vi "运维调试_总磷总氮.vi"() -> ()   [LabVIEW 2016, in "斯坦道氨氮.lvlib"]
uses:
  <vilib>/Utility/miscctls.llb/LVPointTypeDef.ctl
  <vilib>/Plasmionique/MB Master/MB_Master/MB_Master.lvclass
  <vilib>/ptbypt/NI_PtbyPt.lvlib
panel:
  out "seconds since 1Jan1904 2":timestamp
  out "seconds since 1Jan1904":timestamp
  in  "周期设置":bool
  in  "流程操作":bool
  out "消解压力":sgl format="%#.2f kPa"
  out "权限等级":string
  out "总步数":i32
  out "滑动杆":u8(slide) caption="测试进度" scale=0.0..100.0
  out "试剂余量显示":sgl[][](graph)
  in  "仪器校准":bool
  in  "参数查询":bool
  out "简易步骤名称":string
  in  "温度曲线":bool
  in  "试剂余量":bool
  in  "灯值调整":bool
  out "固件版本号":string
  out "模块版本号":string
  out "注射器温度":sgl format="%#.2f ℃"
  out "消解温度":sgl format="%#.2f ℃"
  out "ADC":sgl
  out "F3":sgl format="%#.6f"
  out "F2":sgl format="%#.6f"
  out "F1":sgl format="%#.6f"
  out "F0":sgl format="%#.6f"
  out "运行状态":T1 {"数据时间:" format="%<%y/%m/%d %H:%M:%S>T"; "仪器时间:" format="%<%y/%m/%d %H:%M:%S>T"}
  in  "单选按钮":T2=enum."总氮"
  in  "布尔":bool
  in  "外设固件":bool
  out "字符串 2":string
  in  "数组":string[](array[string])
  in  "返回":bool
  in  "参数设置":bool
  out "集成报警信息":string
  in  "停止":bool
  in  "手动启动":bool
  in  "调试":bool
  out "多列列表框":i32(listbox)
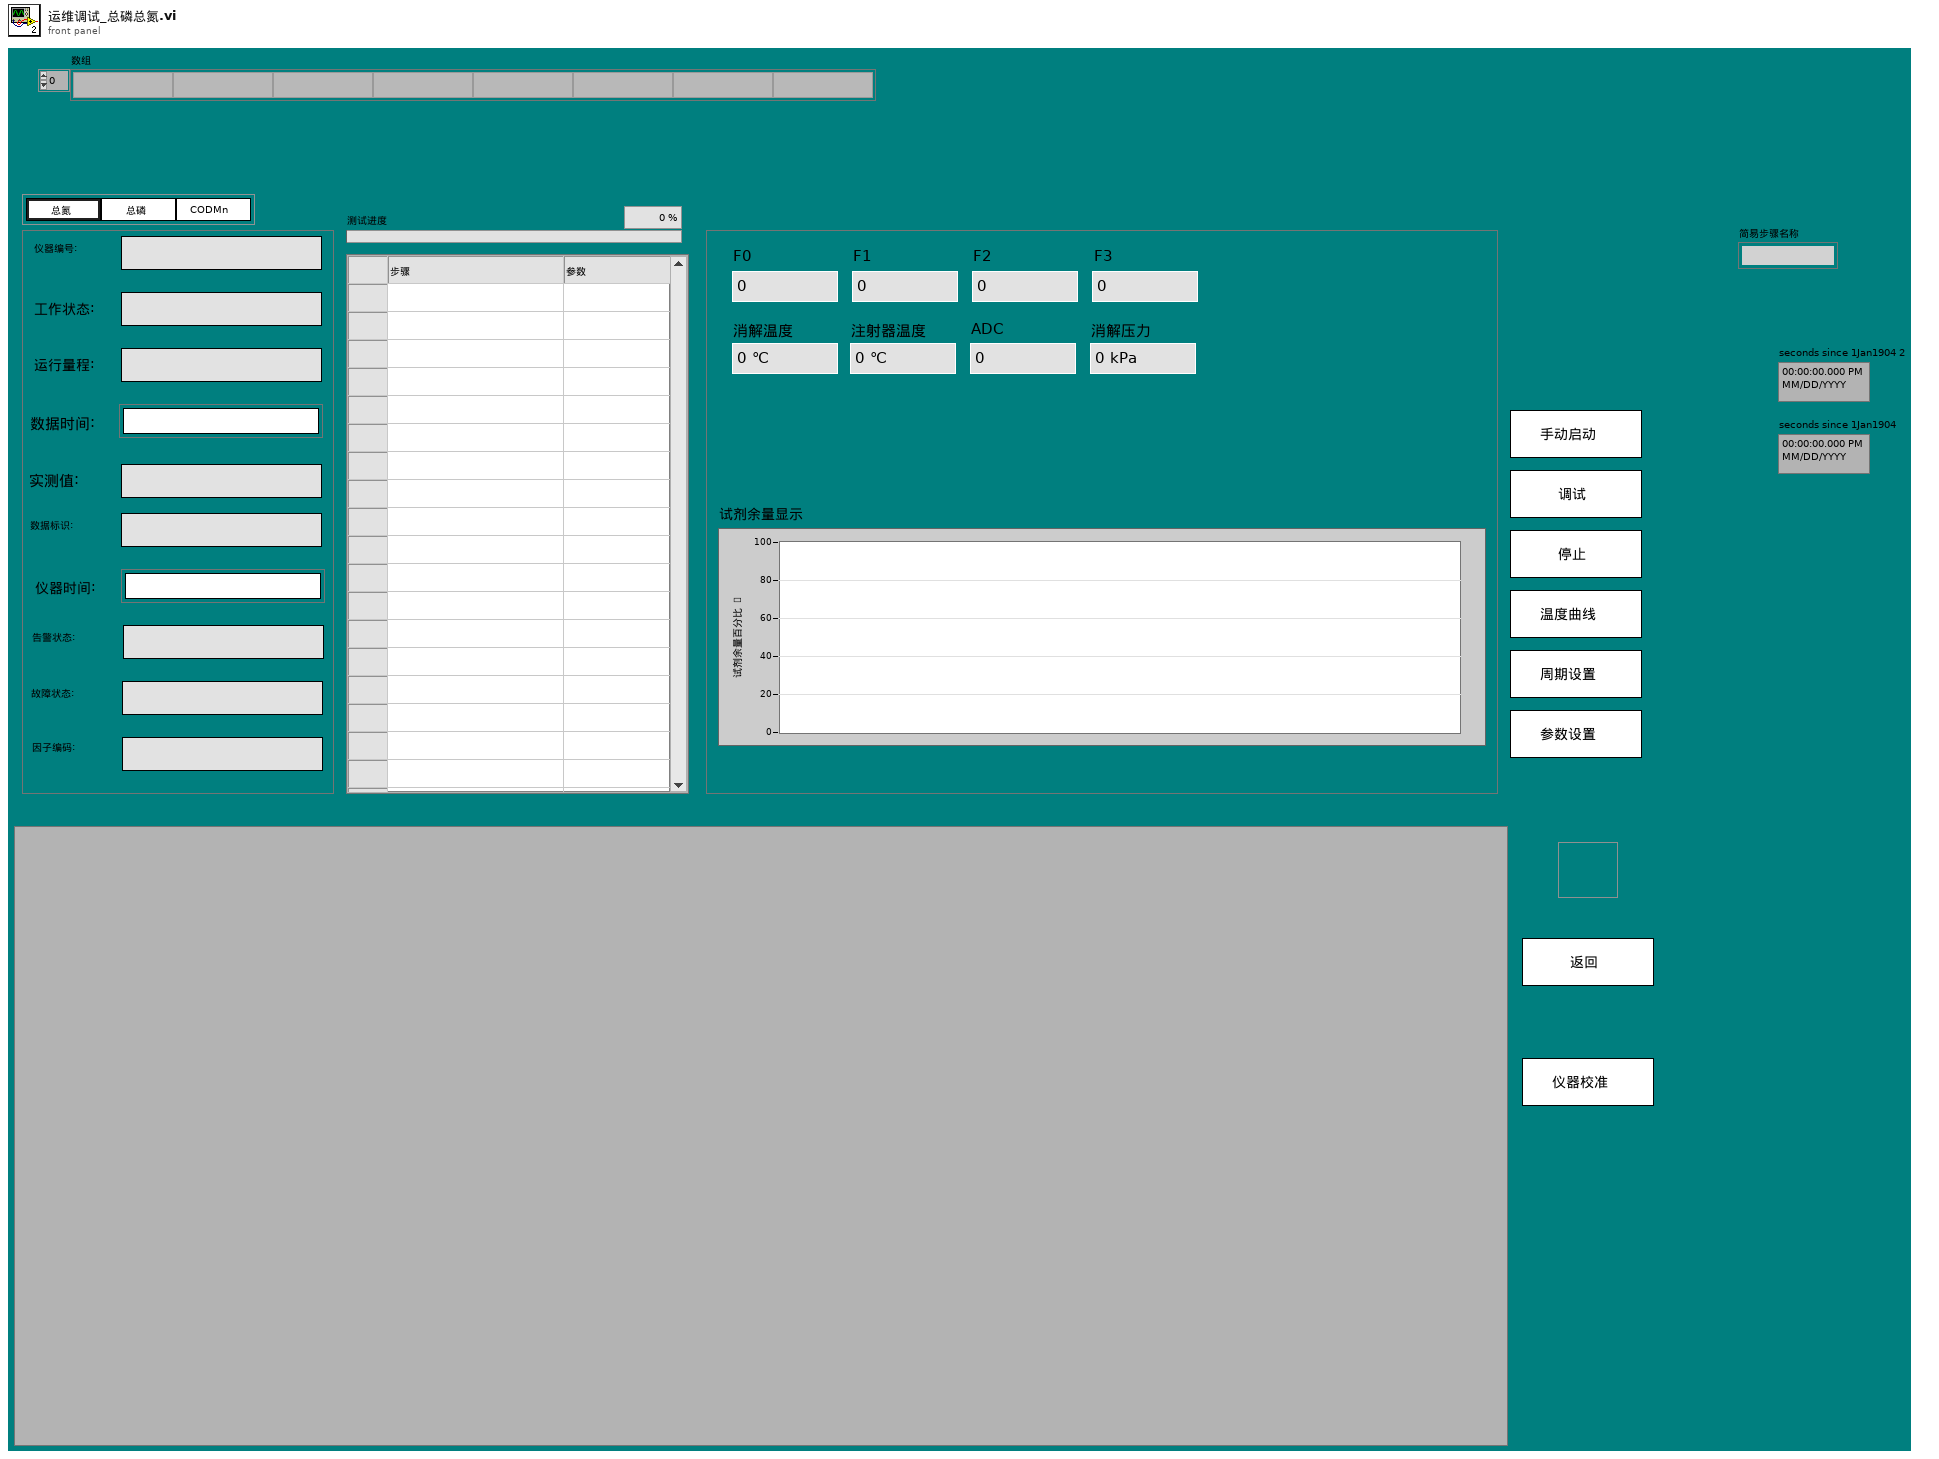
[diagram p1: front panel]
types:
  T1 = cluster{"仪器编号:":string, "工作状态:":string, "运行量程: ":string, "数据时间:":timestamp, "实测值:":string, "数据标识: ":string, "仪器时间:":timestamp, "告警状态: ":string, "故障状态:  ":string, "因子编码:":string}
  T2 = typedef "斯坦道氨氮.lvlib/启动参数显示控件.ctl" = enum32{"COD", "氨氮", "总氮", "总磷", "磷酸盐", "硝氮", "亚硝氮", "硅酸盐", "硫化物", "氟化物", "CODMn"}
  T3 = cluster{"Major":u16, "Minor":u16, "Fix":u16, "Build":u16}
  T4 = typedef "斯坦道总磷总氮.lvlib/启动参数显示控件.ctl" = enum32{"COD", "氨氮", "总氮", "总磷", "磷酸盐", "硝氮", "亚硝氮", "硅酸盐", "硫化物", "氟化物", "CODMn"}
  T5 = typedef "LVPointTypeDef.ctl" = cluster{"Horizontal":i16, "Vertical":i16}
  T6 = cluster{"系统时间":timestamp, "工作状态":u16, "测量模式":enum16{"待机", "连续模式", "周期模式", "定点模式", "受控模式", "手动模式"}, "告警代码":u16, "故障代码":u16, "日志代码":u16, "软件版本":u16, "F0":sgl, "F1":sgl, "F2":sgl, "F3":sgl, "T":sgl, "H":sgl, "id":u16, "flowid":u16, "量程":u16, "总磷控温温度1":sgl, "营养盐控温温度2":sgl, "ADC":sgl}
  T7 = typedef "Alarm interface.lvlib/报警短信语音交互.ctl" = cluster{"参数":string, "元器件":string, "故障现象":string, "code":string, "platform_alarm_code":string, "solutionList":cluster{"reason":string, "solution":string}[]}
  T8 = typedef "SingleStepTestV3.lvlib/SingleStepTestV3.lvclass/仪器版本.ctl" = enum16{"A版", "B版", "A1版"}
  T9 = cluster{"因子编码":u32, "单位":u16, "标样参考值":sgl, "水样数据时间":timestamp, "水样实测值":sgl, "水样数据标识":string, "标样数据时间":timestamp, "标样实测值":sgl, "标样数据标识":string, "空白数据时间":timestamp, "空白实测值":sgl, "空白数据标识":string, "零点核查数据时间":timestamp, "零点核查实测值":sgl, "零点核查数据标识":string, "跨度核查数据时间":timestamp, "跨度核查实测值":sgl, "跨度核查数据标识":string, "加标回收数据时间":timestamp, "加标回收实测值":sgl, "加标回收数据标识":string, "平行样数据时间":timestamp, "平行样实测值":sgl, "平行样数据标识":string, "F0":sgl, "F1":sgl, "F2":sgl, "F3":sgl, "F4":sgl, "F5":sgl, "F6":sgl, "F7":sgl, "温度":sgl, "湿度":sgl, "X值":sgl, "fidrange":u16, "X1值":sgl}[]
  T10 = cluster{"因子编码":u32, "单位":u16, "标样参考值":sgl, "水样数据时间":timestamp, "水样实测值":sgl, "水样数据标识":string, "标样数据时间":timestamp, "标样实测值":sgl, "标样数据标识":string, "空白数据时间":timestamp, "空白实测值":sgl, "空白数据标识":string, "零点核查数据时间":timestamp, "零点核查实测值":sgl, "零点核查数据标识":string, "跨度核查数据时间":timestamp, "跨度核查实测值":sgl, "跨度核查数据标识":string, "加标回收数据时间":timestamp, "加标回收实测值":sgl, "加标回收数据标识":string, "平行样数据时间":timestamp, "平行样实测值":sgl, "平行样数据标识":string, "F0":sgl, "F1":sgl, "F2":sgl, "F3":sgl, "F4":sgl, "F5":sgl, "F6":sgl, "F7":sgl, "温度":sgl, "湿度":sgl, "X值":sgl, "fidrange":u16, "X1值":sgl}
  T11 = typedef "TimingControl.lvlib/TimingControl.lvclass/国标控制命令.ctl" = enum16{"启动测量", "标样核查", "零点核查", "跨度核查", "空白测试", "平行样测试", "加标回收", "空白校准", "标样校准", "初始化（清洗）", "停止测试", "仪器重启", "校时", "模式设置", "测量间隔设置"}
  T12 = typedef "TimingControl.lvlib/TimingControl.lvclass/测量参数.ctl" = u16
  T13 = enum32{"Bad", "Idle", "Run top level", "Running"}
  T14 = enum16{"空闲", "水样测试", "标样核查", "零点核查", "跨度核查", "空白测试", "平行样测试", "加标回收", "空白校准", "标样校准", "初始化（清洗）"}
  T15 = cluster{"站号":u16, "量程切换":enum32{"H", "L", "AUTO"}, "控制命令":enum16{"启动测量", "标样核查", "零点核查", "跨度核查", "空白测试", "平行样测试", "加标回收", "空白校准", "标样校准", "初始化（清洗）", "停止测试", "仪器重启", "校时", "模式设置", "测量间隔设置"}, "模式设置":enum16{"待机", "连续模式", "周期模式", "定点模式", "受控模式", "手动模式"}, "测量间隔":u16}
  T16 = cluster{"时间标识":timestamp, "设备":string, "日志信息":string, "流程参数":string}
  T17 = typedef "LVRowAndColumnUnsignedTypeDef.ctl" = cluster{"Row":u32, "Column":u32}
  T18 = typedef "操作日志字段定义.ctl" = cluster{"时间":timestamp, "参数":string, "日志信息":string, "流程参数":string}
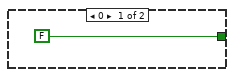
[diagram p4: hidden frame]
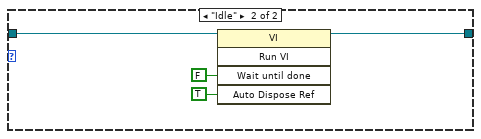
[diagram p8: hidden frame]
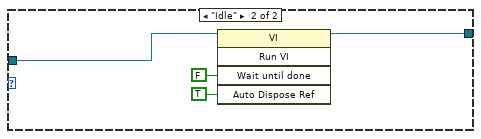
[diagram p9: hidden frame]
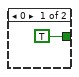
[diagram p11: hidden frame]
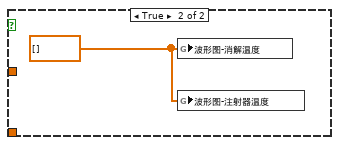
[diagram p12: hidden frame]
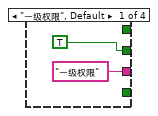
[diagram p14: hidden frame]
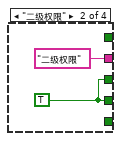
[diagram p15: hidden frame]
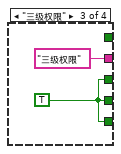
[diagram p16: hidden frame]
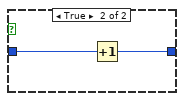
[diagram p18: hidden frame]
diagram:
  n1 = flat-sequence {
    tunnel: [w27] -> w18
    tunnel: w18 -> [w39]
    tunnel: [w39] -> w17
    tunnel: w17 -> [w64]
    tunnel: [w155] -> w19
    tunnel: [errorcluster {"status"=FALSE, "code"=0, "source"=""} ("错误输入（无错误）")] -> w8
    tunnel: [errorcluster {"status"=FALSE, "code"=0, "source"=""} ("错误输入（无错误）")] -> w7
    tunnel: [w152] -> w5
    tunnel: [errorcluster {"status"=FALSE, "code"=0, "source"=""} ("error out")] -> w4
    tunnel: [errorcluster {"status"=FALSE, "code"=0, "source"=""} ("错误输入（无错误）")] -> w3
    frame #0 {
      n2 = control-ref of="本VI"() -> (w29:refnum<vi>)
      n3 = control-ref of="本VI"() -> (w38:refnum<vi>)
      n4 = property class="VI"(reference=w29) -> ("Library"=w30:refnum<vi>)  [unwired: 1 in, 2 out]
      n5 = property class="VI"(reference=w38) -> ("Library.Version"=w37:T3)  [unwired: 1 in, 2 out]
      n6 = global read "VAR总磷总氮全局变量.vi" "初始化"() -> (w26:bool)
      n7 = case shown="假" w26 {
        frame False {
          n8 = call "配置初始化.vi"() -> ()  [unwired: 11 in, 1 out]
        }
        frame True {
        }
      }
      n9 = property class="Library"(reference=w30) -> ("Path"=w28:path)  [unwired: 1 in, 2 out]
      n10 = Unbundle By Name(w37) -> ("Major"=w35:u16, "Minor"=w34:u16, "Fix"=w33:u16, "Build"=w32:u16)
      n11 = call "新建通讯互斥锁.vi"() -> ()  [unwired: 11 in, 1 out]
      n12 = Format Into String(format string="模块版本号：%d.%d.%d.%d" ("格式字符串"), w35, w34, w33, w32) -> (resulting string=→"模块版本号":string)  [unwired: 2 in, 1 out]
      n13 = call <vilib>:"Get File Extension.vi"("file"=w28) -> ("filename without extension"=w27:string)  [unwired: 6 in, 4 out]
    }
    frame #1 {
      n14 = global read "总磷总氮断电保存全局变量.vi" "IP"() -> (w43:string)
      n15 = global read "总磷总氮断电保存全局变量.vi" "VISA Resource"() -> (w40:refnum<visa-resource-name>)
      n16 = Empty String/Path?(string/path=w43) -> (empty?=w42:bool)
      n17 = Empty String/Path?(string/path=w40) -> (empty?=w41:bool)
      n18 = case shown="真" w42 {
        tunnel: w39 -> [_ w55]
        frame False {
        }
        frame True {
          n19 = case shown="\"斯坦道CODMn\"" w55 {
            tunnel: [w56 "192.168.1.203" ("IP") "192.168.1.202" ("IP") "192.168.1.202" ("IP") "192.168.1.203" ("IP") "192.168.1.204" ("IP") "192.168.1.205" ("IP") "192.168.1.201" ("IP")] -> w54
            frame Default {
              n20 = global read "总磷总氮断电保存全局变量.vi" "IP"() -> (w56:string)
            }
            frame "斯坦道总磷总氮" {
            }
            frame "斯坦道氨氮" {
            }
            frame "斯坦道氨氮总磷" {
            }
            frame "斯坦道总磷" {
            }
            frame "斯坦道总氮" {
            }
            frame "斯坦道CODcr" {
            }
            frame "斯坦道CODMn" {
            }
          }
          n21 = global write "总磷总氮断电保存全局变量.vi" "IP"(w54) -> ()
        }
      }
      n22 = case shown="真" w41 {
        tunnel: w39 -> [_ w45]
        frame False {
        }
        frame True {
          n23 = case shown="\"斯坦道CODMn\"" w45 {
            tunnel: [w46 "COM5" ("IP") "COM7" ("IP") "COM7" ("IP") "COM5" ("IP") "COM10" ("IP") "COM9" ("IP") "COM4" ("IP")] -> w44
            frame Default {
              n24 = global read "总磷总氮断电保存全局变量.vi" "VISA Resource"() -> (w46:refnum<visa-resource-name>)
            }
            frame "斯坦道总磷总氮" {
            }
            frame "斯坦道氨氮" {
            }
            frame "斯坦道氨氮总磷" {
            }
            frame "斯坦道总磷" {
            }
            frame "斯坦道总氮" {
            }
            frame "斯坦道CODcr" {
            }
            frame "斯坦道CODMn" {
            }
          }
          n25 = global write "总磷总氮断电保存全局变量.vi" "VISA Resource"(w44) -> ()
        }
      }
    }
    frame #2 {
      n26 = global read "model config var.vi" "启动队列名称"() -> (w66:cluster{"String":string, "Value":u16}[])
      n27 = Empty Array?(array=w66) -> (empty?=w65:bool)
      n28 = case shown="真" w65 {
        tunnel: w64 -> [_ w67]
        frame False {
        }
        frame True {
          n29 = global read "总磷总氮断电保存全局变量.vi" "PORT"() -> (w73:string)
          n30 = Decimal String To Number(string=w73) -> (number=w72:i32)  [unwired: 2 in, 1 out]
          n31 = global read "总磷总氮断电保存全局变量.vi" "MB通信方式选择"() -> (w71:enum16{"串口", "TCP"})
          n32 = global read "总磷总氮断电保存全局变量.vi" "VISA Resource"() -> (w70:refnum<visa-resource-name>)
          n33 = global read "总磷总氮断电保存全局变量.vi" "IP"() -> (w74:string)
          n34 = call "获取启动参数.vi"("MB通信方式选择"=w71, "Port (502)"=w72, "IP Address"=w74, "VISA Resource"=w70) -> ("error out"=w69:errorcluster, "数组"=w68:cluster{"String":string, "Value":u16}[])  [unwired: 6 in]
          n35 = flat-sequence {
            tunnel: w69 -> [w76]
            tunnel: w68 -> [w75]
            tunnel: w67 -> [w78]
            frame #0 {
              n36 = case shown="无错误" w76 {
                tunnel: w75 -> [w77 _]
                frame No Error {
                  n37 = global write "model config var.vi" "启动队列名称"(w77) -> ()
                }
                frame Error {
                }
              }
            }
            frame #1 {
              n38 = global read "model config var.vi" "启动队列名称"() -> (w80:cluster{"String":string, "Value":u16}[])
              n39 = Empty Array?(array=w80) -> (empty?=w79:bool)
              n40 = case shown="真" w79 {
                tunnel: w78 -> [_ w81]
                frame False {
                }
                frame True {
                  n41 = case shown="\"斯坦道CODmn\"" w81 {
                    frame Default {
                    }
                    frame "斯坦道总磷总氮" {
                      n42 = global write "model config var.vi" "启动队列名称"(cluster{"String":string, "Value":u16}[] [{"String"="总氮", "Value"=2}, {"String"="总磷", "Value"=1}] ("启动队列名称")) -> ()
                    }
                    frame "斯坦道氨氮" {
                      n43 = global write "model config var.vi" "启动队列名称"(cluster{"String":string, "Value":u16}[] [{"String"="氨氮", "Value"=3}] ("启动队列名称")) -> ()
                    }
                    frame "斯坦道氨氮总磷" {
                      n44 = global write "model config var.vi" "启动队列名称"(cluster{"String":string, "Value":u16}[] [{"String"="氨氮", "Value"=3}, {"String"="总磷", "Value"=1}] ("启动队列名称")) -> ()
                    }
                    frame "斯坦道总磷" {
                      n45 = global write "model config var.vi" "启动队列名称"(cluster{"String":string, "Value":u16}[] [{"String"="总磷", "Value"=1}] ("启动队列名称")) -> ()
                    }
                    frame "斯坦道总氮" {
                      n46 = global write "model config var.vi" "启动队列名称"(cluster{"String":string, "Value":u16}[] [{"String"="总氮", "Value"=2}] ("启动队列名称")) -> ()
                    }
                    frame "斯坦道CODcr" {
                      n47 = global write "model config var.vi" "启动队列名称"(cluster{"String":string, "Value":u16}[] [{"String"="CODcr", "Value"=22}] ("启动队列名称")) -> ()
                    }
                    frame "斯坦道氟化物" {
                      n48 = global write "model config var.vi" "启动队列名称"(cluster{"String":string, "Value":u16}[] [{"String"="氟化物", "Value"=50}] ("启动队列名称")) -> ()
                    }
                    frame "斯坦道CODmn" {
                      n49 = global write "model config var.vi" "启动队列名称"(cluster{"String":string, "Value":u16}[] [{"String"="CODMn", "Value"=21}] ("启动队列名称")) -> ()
                    }
                  }
                }
              }
            }
            frame #2 {
              n50 = call "模块配置写入.vi"() -> ()  [unwired: 11 in, 1 out]
            }
          }
        }
      }
    }
    frame #3 {
      # "初始化"
      n51 = global read "总磷总氮断电保存全局变量.vi" "流程路径"() -> (w94:path)
      n52 = global read "model config var.vi" "启动队列名称"() -> (w100:cluster{"String":string, "Value":u16}[])
      n53 = global read "总磷总氮断电保存全局变量.vi" "简易流程路径"() -> (w91:path)
      n54 = call <vilib>:"Check if File or Folder Exists.vi"("path"=w94) -> ("file or folder exists?"=w99:bool)  [unwired: 8 in, 2 out]
      n55 = for {
        tunnel: w100 -> [w117] mode=indexing
        shift-right: [w116] -> w101
        shift-left: "" -> [w114]
        n56 = Unbundle By Name(w117) -> ("String"=w115:string)
        n57 = Concatenate Strings(w114, w115) -> (w116:string)
      }
      n58 = call <vilib>:"Check if File or Folder Exists.vi"("path"=w91) -> ("file or folder exists?"=w98:bool)  [unwired: 8 in, 2 out]
      n59 = Empty String/Path?(string/path=w94) -> (empty?=w95:bool)
      n60 = Not(x=w99) -> (.not. x?=w97:bool)
      n61 = Empty String/Path?(string/path=w91) -> (empty?=w90:bool)
      n62 = Not(x=w98) -> (.not. x?=w93:bool)
      n63 = Or(x=w95, y=w97) -> (x .or. y?=w96:bool)
      n64 = Or(x=w90, y=w93) -> (x .or. y?=w92:bool)
      n65 = case shown="真" w96 {
        frame False {
        }
        frame True {
          n66 = global read "model config var.vi" "启动队列名称"() -> (w110:cluster{"String":string, "Value":u16}[])
          n67 = for {
            tunnel: w110 -> [w113] mode=indexing
            tunnel: [w112] -> w109 mode=indexing
            n68 = Unbundle By Name(w113) -> ("String"=w112:string)
          }
          n69 = call "获取默认流程路径.vi"("参数"=w109) -> ("路径"=w111:path)  [unwired: 10 in]
          n70 = global write "总磷总氮断电保存全局变量.vi" "流程路径"(w111) -> ()
        }
      }
      n71 = case shown="真" w92 {
        frame False {
        }
        frame True {
          n72 = global read "model config var.vi" "启动队列名称"() -> (w105:cluster{"String":string, "Value":u16}[])
          n73 = for {
            tunnel: w105 -> [w108] mode=indexing
            tunnel: [w107] -> w104 mode=indexing
            n74 = Unbundle By Name(w108) -> ("String"=w107:string)
          }
          n75 = call "获取默认流程路径.vi"("复合步骤"=TRUE, "参数"=w104) -> ("路径"=w106:path)  [unwired: 9 in]
          n76 = global write "总磷总氮断电保存全局变量.vi" "简易流程路径"(w106) -> ()
        }
      }
      n77 = global write "VAR总磷总氮全局变量.vi" "模块名称"(w101) -> ()
    }
    frame #4 {
      n78 = global read "model config var.vi" "启动队列名称"() -> (w120:cluster{"String":string, "Value":u16}[])
      n79 = vi-ref "总磷总氮测量数据储存.vi"() -> (w130:refnum<vi>)
      n80 = vi-ref "总磷总氮通讯.vi"() -> (w122:refnum<vi>)
      n81 = Index Array(array=w120) -> (element=w119:cluster{"String":string, "Value":u16})  [unwired: 1 in]
      n82 = property class="VI"(reference=w130) -> ("Name"=w137:string)  [unwired: 1 in, 2 out]
      n83 = property class="VI"(reference=w122) -> ("Name"=w123:string)  [unwired: 1 in, 2 out]
      n84 = Unbundle By Name(w119) -> ("Value"=w118:u16)
      n85 = case shown="50" w118 {
        tunnel: [w138 启动参数显示控件."总磷" ("单选按钮") 启动参数显示控件."总氮" ("单选按钮") 启动参数显示控件."COD" ("单选按钮") 启动参数显示控件."氨氮" ("单选按钮") 启动参数显示控件."磷酸盐" ("单选按钮") 启动参数显示控件."硝氮" ("单选按钮") 启动参数显示控件."亚硝氮" ("单选按钮") 启动参数显示控件."硅酸盐" ("单选按钮") 启动参数显示控件."硫化物" ("单选按钮") 启动参数显示控件."氟化物" ("单选按钮") 启动参数显示控件."CODMn" ("单选按钮")] -> w121
        frame 0, Default {
          n86 = property on="单选按钮" class="RadioBtnsControl (严格)"() -> ("Value"=w138:T4)  [unwired: 2 in, 2 out]
        }
        frame 1 {
        }
        frame 2 {
        }
        frame 22 {
        }
        frame 3 {
        }
        frame 4 {
        }
        frame 5 {
        }
        frame 6 {
        }
        frame 7 {
        }
        frame 8 {
        }
        frame 50 {
        }
        frame 21 {
        }
      }
      n87 = Open VI Reference(type specifier VI Refnum (for type only)=refnum<vi> refnum, vi path=w137, options=128 ("选项")) -> (vi reference=w135:refnum<vi>, error out=w133:errorcluster)  [unwired: 3 in]
      n88 = Open VI Reference(type specifier VI Refnum (for type only)=refnum<vi> refnum, vi path=w123, options=128 ("选项")) -> (vi reference=w125:refnum<vi>, error out=w127:errorcluster)  [unwired: 3 in]
      n89 = call-by-ref "开始异步调用"(reference=w135, error in=w133) -> (reference out=w131:refnum<vi>, error out=w132:errorcluster)  [unwired: 12 in]
      n90 = call-by-ref "开始异步调用"(reference=w125, error in=w127) -> (reference out=w129:refnum<vi>, error out=w128:errorcluster)  [unwired: 12 in]
      n91 = Close Reference(reference=w131, error in (no error)=w132) -> ()  [unwired: 1 out]
      n92 = Close Reference(reference=w129, error in (no error)=w128) -> ()  [unwired: 1 out]
      n93 = property on="单选按钮" class="RadioBtnsControl (严格)"("Value"=w121) -> ()  [unwired: 2 in, 2 out]
    }
    frame #5 {
      n94 = call "配置文件路径.vi"() -> ("appended path"=w152:path)  [unwired: 11 in]
      n95 = call "设置模块队列名.vi"() -> ("Msg"=w155:string)  [unwired: 5 in]
    }
  }
  n96 = flat-sequence {
    frame #0 {
      n97 = property on="窗格" class="Pane"("Origin"=T5 {"Horizontal"=0, "Vertical"=0} ("原点")) -> ()  [unwired: 2 in, 2 out]
    }
  }
  n98 = while {
    stop <- FALSE stop-if-true
    n99 = global read "VAR总磷总氮全局变量.vi" "状态告警区"() -> (w161:T6)
    n100 = Unbundle By Name(w161) -> ("工作状态"=w159:u16)
    n101 = Equal To 0?(x=w159) -> (x = 0?=w158:bool)
    n102 = global read "VAR总磷总氮全局变量.vi" "通讯状态"() -> (w162:bool)
    n103 = And(x=w158, y=w162) -> (x .and. y?=w160:bool)
    n104 = call <vilib>:"Boolean Crossing PtByPt.vi"("input"=w160) -> ("crossing"=w157:bool)  [unwired: 2 in]
    n105 = case shown="真" w157 {
      frame False {
      }
      frame True {
        n106 = control-ref of="试剂余量显示"() -> (w165:refnum<vi>)
        n107 = call "试剂余量展示.vi"("波形图 2"=w165) -> ("波形图"=→"试剂余量显示":sgl[][])  [unwired: 10 in]
      }
    }
    n108 = Wait (ms)(milliseconds to wait=u32 1000 ("等待时间（毫秒）")) -> ()  [unwired: 1 out]
  }
  n109 = while {
    shift-right: [w176] -> _
    shift-left: u32 0 ("y") -> [w178]
    stop <- FALSE stop-if-true
    # "密码权限"
    n110 = global read "VAR总磷总氮全局变量.vi" "权限等级"() -> (w173:enum16{"一级权限", "二级权限", "三级权限", "超级权限"})
    n111 = case shown="\"超级权限\"" w173 {
      tunnel: [_ w183 w185 w188] -> w167
      tunnel: [_ _ w185 w188] -> _
      tunnel: [_ w183 w185 w188] -> w172
      tunnel: [_ _ _ TRUE] -> _
      tunnel: [TRUE _ _ _] -> w170
      tunnel: ["一级权限" "二级权限" "三级权限" "超级权限"] -> w168
      frame "一级权限", Default {
      }
      frame "二级权限" {
        w183 = TRUE
      }
      frame "三级权限" {
        w185 = TRUE
      }
      frame "超级权限" {
        w188 = TRUE
      }
    }
    "权限等级" <- w168
    n112 = case shown="假" "布尔" {
      tunnel: w178 -> [_ w191]
      tunnel: [_ w190] -> w176
      frame False {
      }
      frame True {
        n113 = Increment(x=w191) -> (x+1=w190:u32)
      }
    }
    n114 = Wait (ms)(milliseconds to wait=u32 1000 ("等待时间（毫秒）")) -> ()  [unwired: 1 out]
    n115 = Not(x=w170) -> (.not. x?=w169:bool)
    n116 = property on="外设固件" class="Bool"("Visible"=w172) -> ()  [unwired: 2 in, 2 out]
    n117 = property on="流程操作" class="Bool"("Visible"=w167) -> ()  [unwired: 2 in, 2 out]
    n118 = property on="试剂余量" class="Bool"("Visible"=w167) -> ()  [unwired: 2 in, 2 out]
    n119 = property on="灯值调整" class="Bool"("Visible"=w167) -> ()  [unwired: 2 in, 2 out]
    n120 = Greater Or Equal?(x=w176, y=u32 3600) -> (x >= y?=w174:bool)
    n121 = property on="布尔" class="Bool (严格)"("Value"=w169) -> ()  [unwired: 2 in, 2 out]
    n122 = case shown="真" w174 {
      frame False {
      }
      frame True {
        n123 = global write "VAR总磷总氮全局变量.vi" "权限等级"(enum16{"一级权限", "二级权限", "三级权限", "超级权限"}."一级权限" ("权限等级")) -> ()
      }
    }
  }
  n124 = while {
    shift-right: [w204] -> _
    shift-left: u16 1 ("工作状态") -> [w202]
    stop <- FALSE stop-if-true
    (unwired) "注射器温度"
    n125 = global read "VAR总磷总氮全局变量.vi" "状态告警区"() -> (w224:T6)
    n126 = global read "VAR总磷总氮全局变量.vi" "通讯状态"() -> (w235:bool)
    n127 = global read "VAR总磷总氮全局变量.vi" "状态告警区"() -> (w233:T6)
    n128 = global write "VAR总磷总氮全局变量.vi" "最近一次工作状态"(w202) -> ()
    n129 = Unbundle By Name(w224) -> ("id"=w223:u16, "工作状态"=w219:u16)
    n130 = case shown="真" w235 {
      tunnel: ["通讯异常" ("集成报警信息") w354] -> w234
      frame False {
      }
      frame True {
        n131 = global read "VAR总磷总氮全局变量.vi" "状态告警区"() -> (w356:T6)
        n132 = local read "seconds since 1Jan1904 2"() -> (w346:timestamp)
        n133 = local read "seconds since 1Jan1904"() -> (w349:timestamp)
        n134 = Subtract(x=w346, y=w349) -> (x-y=w345:dbl)
        n135 = Unbundle By Name(w356) -> ("工作状态"=w352:u16)
        n136 = Not Equal To 0?(x=w352) -> (x != 0?=w348:bool)
        n137 = Get Date/Time In Seconds() -> (seconds since 1Jan1904=w347:timestamp)
        n138 = global read "VAR总磷总氮全局变量.vi" "测量状态"() -> (w353:string)
        n139 = Greater Or Equal?(x=w345, y=36000.0) -> (x >= y?=w342:bool)
        n140 = case shown="真" w348 {
          tunnel: w347 -> [_ w357]
          frame False {
          }
          frame True {
            "seconds since 1Jan1904 2" <- w357
          }
        }
        n141 = Format Into String(format string="工作计时: %d 秒" ("格式字符串"), initial string=w353, w345) -> (resulting string=w354:string)  [unwired: 1 in, 1 out]
        n142 = call <vilib>:"Boolean Crossing PtByPt.vi"("direction"=enum16{"either", "false-true", "true-false"}."false-true", "input"=w348) -> ("crossing"=w350:bool)  [unwired: 1 in]
        n143 = Or(x=w350, y=w342) -> (x .or. y?=w343:bool)
        n144 = case shown="真" w343 {
          tunnel: w347 -> [_ w358]
          frame False {
          }
          frame True {
            "seconds since 1Jan1904" <- w358
          }
        }
      }
    }
    "集成报警信息" <- w234
    n145 = Unbundle By Name(w233) -> ("flowid"=w201:u16, "系统时间"=w229:timestamp, "工作状态"=w228:u16, "告警代码"=w222:u16, "故障代码"=w221:u16, "量程"=w227:u16)
    n146 = case shown="\"磷酸盐\"" "单选按钮" {
      tunnel: [22 3 2 1 4 5 6 7 8 50 21] -> w192
      tunnel: [_ TRUE _ _ _ _ _ _ _ _ _] -> w196
      frame "COD", Default {
      }
      frame "氨氮" {
      }
      frame "总氮" {
      }
      frame "总磷" {
      }
      frame "磷酸盐" {
      }
      frame "硝氮" {
      }
      frame "亚硝氮" {
      }
      frame "硅酸盐" {
      }
      frame "硫化物" {
      }
      frame "氟化物" {
      }
      frame "CODMn" {
      }
    }
    n147 = First Call?() -> (First Call?: T/F=w193:bool)
    n148 = case shown="1, 默认" w219 {
      tunnel: w223 -> [_ w291]
      frame 0 {
      }
      frame 1, Default {
        n149 = case shown="21" w291 {
          tunnel: [w292 启动参数显示控件."总磷" ("单选按钮") 启动参数显示控件."总氮" ("单选按钮") 启动参数显示控件."COD" ("单选按钮") 启动参数显示控件."氨氮" ("单选按钮") 启动参数显示控件."磷酸盐" ("单选按钮") 启动参数显示控件."硝氮" ("单选按钮") 启动参数显示控件."亚硝氮" ("单选按钮") 启动参数显示控件."硅酸盐" ("单选按钮") 启动参数显示控件."硫化物" ("单选按钮") 启动参数显示控件."CODMn" ("单选按钮") 启动参数显示控件."氟化物" ("单选按钮")] -> w290
          frame 0, Default {
            n150 = property on="单选按钮" class="RadioBtnsControl (严格)"() -> ("Value"=w292:T4)  [unwired: 2 in, 2 out]
          }
          frame 1 {
          }
          frame 2 {
          }
          frame 22 {
          }
          frame 3 {
          }
          frame 4 {
          }
          frame 5 {
          }
          frame 6 {
          }
          frame 7 {
          }
          frame 8 {
          }
          frame 21 {
          }
          frame 50 {
          }
        }
        n151 = property on="单选按钮" class="RadioBtnsControl (严格)"("Value"=w290) -> ()  [unwired: 2 in, 2 out]
      }
    }
    n152 = case shown="2" w228 {
      selector: w228 -> [w308 _ w314 w318 w321 w323 w325 w327 w329 w331 w333 w335 w337 w340]
      tunnel: [w309 "空闲" ("工作状态") "水样测量" ("工作状态") w317 "零点核查" ("工作状态") "跨度核查" ("工作状态") "空白测试" ("工作状态") "平行样测试" ("工作状态") "加标回收" ("工作状态") "空白校准" ("工作状态") "标样校准" ("工作状态") "初始化" ("工作状态") "单步调试" ("工作状态") w339] -> w203
      tunnel: [w307 w312 w314 w318 w321 w323 w325 w327 w329 w331 w333 w335 w337 w340] -> w204
      tunnel: w202 -> [w307 w312 _ _ _ _ _ _ _ _ _ _ _ _]
      tunnel: w201 -> [_ _ _ w316 _ _ _ _ _ _ _ _ _ _]
      frame Default {
        n153 = Format Into String(format string="%d" ("格式字符串"), initial string="未知" ("工作状态"), w308) -> (resulting string=w309:string)  [unwired: 1 in, 1 out]
      }
      frame 0 {
      }
      frame 1 {
      }
      frame 2 {
        n154 = case shown="5" w316 {
          tunnel: ["标样核查" ("工作状态") "快捷测试" ("工作状态")] -> w317
          frame 0, Default {
          }
          frame 5 {
          }
        }
      }
      frame 3 {
      }
      frame 4 {
      }
      frame 5 {
      }
      frame 6 {
      }
      frame 7 {
      }
      frame 8 {
      }
      frame 9 {
      }
      frame 10 {
      }
      frame 254 {
      }
      frame 255 {
        n155 = local read "简易步骤名称"() -> (w339:string)
      }
    }
    n156 = call "告警码字段定义.vi"("id"=w192, "首次调用？"=w193, "告警代码"=w222) -> ("告警信息"=w200:T7)  [unwired: 8 in]
    n157 = call "故障码字段定义.vi"("id"=w192, "首次调用？"=w193, "故障代码"=w221) -> ("告警信息"=w220:T7)  [unwired: 8 in]
    n158 = case shown="1" w227 {
      tunnel: ["" ("字符串") "低量程 " ("字符串") "高量程 " ("字符串")] -> w226
      frame Default {
      }
      frame 0 {
      }
      frame 1 {
      }
    }
    n159 = Unbundle By Name(w200) -> ("故障现象"=w199:string)
    n160 = Unbundle By Name(w220) -> ("故障现象"=w194:string)
    n161 = call "id参数转换.vi"("id"=w192) -> ("数组资源索引"=w205:i32)  [unwired: 9 in, 1 out]
    n162 = call "版本判断.vi"() -> ("仪器版本"=w198:T8)  [unwired: 11 in]
    n163 = global read "VAR总磷总氮全局变量.vi" "测量数据区数组"() -> (w208:T9)
    n164 = case shown="\"A版\", 默认" w198 {
      tunnel: [w238 "传感器" ("标题.文本")] -> w195
      tunnel: ["%#.2f ℃" ("数值文本.格式字符串") "%#.2f " ("数值文本.格式字符串")] -> w197
      tunnel: w196 -> [w241 _]
      frame "A版", Default {
        n165 = Select(t="显色温度", s=w241, f="注射器温度" ("标题.文本")) -> (s? t:f=w238:string)
      }
      frame "B版" {
      }
    }
    n166 = Index Array(array=w208, index=w205) -> (element=w207:T10)
    n167 = case shown="0, 默认" w202 {
      tunnel: [w259 w265 w269 w273 w277 w281 w285 w289] -> w218
      tunnel: [w257 w264 w268 w272 w275 w280 w284 w288] -> w213
      tunnel: [w260 w263 w267 w271 w274 w279 w283 w287] -> w211
      tunnel: w207 -> [_ w262 w266 w270 w276 w278 w282 w286]
      frame 0, Default {
        n168 = local read "运行状态"() -> (w261:T1)
        n169 = Unbundle By Name(w261) -> ("数据时间:"=w259:timestamp, "实测值:"=w258:string, "数据标识:"=w260:string)
        n170 = Fract/Exp String To Number(string=w258) -> (number=w257:dbl)  [unwired: 3 in, 1 out]
      }
      frame 1 {
        n171 = Unbundle By Name(w262) -> ("水样数据时间"=w265:timestamp, "水样实测值"=w264:sgl, "水样数据标识"=w263:string)
      }
      frame 2, 9 {
        n172 = Unbundle By Name(w266) -> ("标样数据时间"=w269:timestamp, "标样实测值"=w268:sgl, "标样数据标识"=w267:string)
      }
      frame 3 {
        n173 = Unbundle By Name(w270) -> ("零点核查数据时间"=w273:timestamp, "零点核查实测值"=w272:sgl, "零点核查数据标识"=w271:string)
      }
      frame 4 {
        n174 = Unbundle By Name(w276) -> ("跨度核查数据时间"=w277:timestamp, "跨度核查实测值"=w275:sgl, "跨度核查数据标识"=w274:string)
      }
      frame 7 {
        n175 = Unbundle By Name(w278) -> ("加标回收数据时间"=w281:timestamp, "加标回收实测值"=w280:sgl, "加标回收数据标识"=w279:string)
      }
      frame 5, 8 {
        n176 = Unbundle By Name(w282) -> ("空白数据时间"=w285:timestamp, "空白实测值"=w284:sgl, "空白数据标识"=w283:string)
      }
      frame 6 {
        n177 = Unbundle By Name(w286) -> ("平行样数据时间"=w289:timestamp, "平行样实测值"=w288:sgl, "平行样数据标识"=w287:string)
      }
    }
    n178 = Unbundle By Name(w207) -> ("因子编码"=w209:u32)
    n179 = global write "VAR总磷总氮全局变量.vi" "工作状态:"(w203) -> ()
    n180 = Format Into String(format string="w%05d" ("格式字符串"), w209) -> (resulting string=w225:string)  [unwired: 2 in, 1 out]
    n181 = property on="注射器温度" class="DigNum (严格)"("Caption.Text"=w195, "NumText.FormatString"=w197) -> ()  [unwired: 2 in, 2 out]
    n182 = Wait (ms)(milliseconds to wait=u32 1000 ("等待时间（毫秒）")) -> ()  [unwired: 1 out]
    n183 = Number To Fractional String(number=w213, precision (6)=i16 4 ("精度(6)")) -> (F-format string=w215:string)  [unwired: 2 in]
    n184 = Concatenate Strings(w215, " " ("字符串"), "mg/L" ("字符串")) -> (w212:string)
    n185 = global read "VAR总磷总氮全局变量.vi" "序列号"() -> (w230:string)
    n186 = Bundle By Name(cluster=T1 {"仪器编号:"="", "工作状态:"="", "运行量程: "="", "数据时间:"=timestamp(0 s since 1904-01-01), "实测值:"="", "数据标识: "="", "仪器时间:"=timestamp(0 s since 1904-01-01), "告警状态: "="", "故障状态:  "="", "因子编码:"=""} ("运行状态"), "仪器编号:"=w230, "仪器时间:"=w229, "工作状态:"=w203, "告警状态:"=w199, "故障状态:"=w194, "运行量程:"=w226, "数据时间:"=w218, "实测值:"=w212, "数据标识:"=w211, "因子编码:"=w225) -> (→"运行状态":T1)
  }
  n187 = while {
    shift-right: [w363] -> _
    shift-left: 0 -> [w364]
    stop <- FALSE stop-if-true
    n188 = global read "VAR总磷总氮全局变量.vi" "心跳包打开状态"() -> (w359:bool)
    n189 = case shown="假" w359 {
      tunnel: w364 -> [w368 _]
      tunnel: [w367 _] -> w363
      frame False {
        n190 = Increment(x=w368) -> (x+1=w367:i32)
      }
      frame True {
      }
    }
    n191 = Wait (ms)(milliseconds to wait=u32 1000 ("等待时间（毫秒）")) -> ()  [unwired: 1 out]
    n192 = Greater Or Equal?(x=w363, y=600) -> (x >= y?=w361:bool)
    n193 = case shown="真" w361 {
      frame False {
      }
      frame True {
        n194 = global write "VAR总磷总氮全局变量.vi" "升级固件关闭心跳包"(FALSE ("关闭心跳包")) -> ()
      }
    }
  }
  n195 = while {
    shift-right: [w370] -> _
    shift-left: TRUE -> [w371]
    stop <- FALSE stop-if-true
    n196 = global read "VAR总磷总氮全局变量.vi" "状态告警区"() -> (w374:T6)
    n197 = global read "VAR总磷总氮全局变量.vi" "状态告警区"() -> (w377:T6)
    n198 = Unbundle By Name(w374) -> ("总磷控温温度1"=w373:sgl)
    n199 = Unbundle By Name(w377) -> ("工作状态"=w372:u16, "总磷控温温度1"=w376:sgl, "营养盐控温温度2"=w375:sgl)
    n200 = call "消解压力计算.vi"("当前消解温度"=w373) -> ("消解压力"=→"消解压力":dbl)  [unwired: 10 in]
    n201 = case shown="1, 默认" w372 {
      tunnel: w376 -> [_ w383]
      tunnel: w375 -> [_ w382]
      tunnel: w371 -> [_ w381]
      tunnel: [TRUE _] -> w370
      frame 0 {
      }
      frame 1, Default {
        n202 = case shown="假" w381 {
          tunnel: w383 -> [w389 _]
          tunnel: w382 -> [w388 _]
          frame False {
            n203 = global read "VAR总磷总氮全局变量.vi" "波形图-消解温度"() -> (w387:sgl[])
            n204 = global read "VAR总磷总氮全局变量.vi" "波形图-注射器温度"() -> (w386:sgl[])
            n205 = Build Array (concatenate)(w387, w389) -> (w385:sgl[])
            n206 = Build Array (concatenate)(w386, w388) -> (w384:sgl[])
            n207 = global write "VAR总磷总氮全局变量.vi" "波形图-消解温度"(w385) -> ()
            n208 = global write "VAR总磷总氮全局变量.vi" "波形图-注射器温度"(w384) -> ()
          }
          frame True {
            w390 = dbl[] [] ("波形图-消解温度")
            n209 = global write "VAR总磷总氮全局变量.vi" "波形图-消解温度"(w390) -> ()
            n210 = global write "VAR总磷总氮全局变量.vi" "波形图-注射器温度"(w390) -> ()
          }
        }
      }
    }
    n211 = Wait (ms)(milliseconds to wait=u32 1000 ("等待时间（毫秒）")) -> ()  [unwired: 1 out]
  }
  n212 = while {
    shift-right: [w391] -> _
    shift-left: _ -> [w396]
    tunnel: w5 -> [w394]
    stop <- FALSE stop-if-true
    n213 = File/Directory Info(path=w394) -> (last mod=w391:timestamp, error out=w392:errorcluster)  [unwired: 1 in, 5 out]
    n214 = Not Equal?(x=w396, y=w391) -> (x != y?=w395:bool)
    n215 = case shown="真" w395 {
      tunnel: [_ w398] -> _
      tunnel: w392 -> [_ _]
      frame False {
      }
      frame True {
        n216 = call "配置初始化.vi"() -> ("error out"=w398:errorcluster)  [unwired: 11 in]
      }
    }
    n217 = Wait (ms)(milliseconds to wait=u32 1000 ("等待时间（毫秒）")) -> ()  [unwired: 1 out]
  }
  n218 = flat-sequence {
    tunnel: w4 -> [_]
    frame #0 {
      n219 = control-ref of="周期设置"() -> (w403:refnum<vi>)
      n220 = call "New TimingControl.vi"("Reference"=w403) -> ("error out"=w401:errorcluster, "TimingControl out"=w402:refnum<class "TimingControl.lvclass">)  [unwired: 9 in]
      n221 = call "taskqueue ref.vi"() -> ("队列输出"=w405:refnum<queue>)  [unwired: 10 in, 1 out]
      n222 = while {
        tunnel: w405 -> [w423]
        shift-right: [w419] -> _
        shift-left: u32 0 ("等待时间（毫秒）") -> [w417]
        shift-right: [w407] -> w400
        shift-left: w402 -> [w412]
        shift-right: [w406] -> w399
        shift-left: w401 -> [w411]
        stop <- FALSE stop-if-true
        n223 = global read "VAR总磷总氮全局变量.vi" "状态告警区"() -> (w425:T6)
        n224 = Unbundle By Name(w425) -> ("工作状态"=w422:u16, "系统时间"=w409:timestamp)
        n225 = Quotient & Remainder(x=w417, y=u32 30) -> (x-y*floor(x/y)=w415:u32)  [unwired: 1 out]
        n226 = Equal To 0?(x=w415) -> (x = 0?=w414:bool)
        n227 = case shown="1, 默认" w422 {
          tunnel: [FALSE TRUE] -> w408
          frame 0 {
          }
          frame 1, Default {
          }
        }
        n228 = Increment(x=w417) -> (x+1=w421:u32)
        n229 = Wait (ms)(milliseconds to wait=u32 500 ("等待时间（毫秒）")) -> ()  [unwired: 1 out]
        n230 = property class="TimingControl"(reference=w412, error in=w411, "Properties:仪器时间"=w409, "Properties:仪器运行状态"=w408) -> (reference out=w407:refnum<class "TimingControl.lvclass">, error out=w406:errorcluster, "Properties:命令输出"=w410:cluster{"启动":bool, "控制命令":T11, "测量参数":T12})
        n231 = Unbundle By Name(w410) -> ("启动"=w418:bool, "控制命令"=w424:T11)
        n232 = And(x=w418, y=w414) -> (x .and. y?=w413:bool)
        n233 = Select(t=w421, s=w418, f=u32 0 ("等待时间（毫秒）")) -> (s? t:f=w419:u32)
        n234 = case shown="真" w413 {
          tunnel: w424 -> [_ w429]
          tunnel: w423 -> [_ w432]
          frame False {
          }
          frame True {
            n235 = Get Queue Status(queue=w432) -> (queue out=w430:refnum<queue>, # elements in queue=w431:i32)  [unwired: 2 in, 6 out]
            n236 = Equal To 0?(x=w431) -> (x = 0?=w428:bool)
            n237 = case shown="真" w428 {
              tunnel: w430 -> [_ w434]
              tunnel: w429 -> [_ w433]
              frame False {
              }
              frame True {
                n238 = Enqueue Element(queue=w434, element=w433) -> ()  [unwired: 2 in, 3 out]
              }
            }
          }
        }
      }
      n239 = call "试剂余量后台任务.vi"() -> ()  [unwired: 12 in]
      n240 = call "task.vi"() -> ()  [unwired: 12 in]
      n241 = call "Close TimingControl.vi"("error in (no error)"=w399, "TimingControl in"=w400) -> ()  [unwired: 9 in, 1 out]
    }
  }
  n242 = while {
    tunnel: w4 -> [_]
    stop <- FALSE stop-if-true
    n243 = flat-sequence {
      frame #0 {
        n244 = global read "model config var.vi" "启动队列名称"() -> (w438:cluster{"String":string, "Value":u16}[])
        n245 = for {
          tunnel: w438 -> [w446] mode=indexing
          shift-right: [w445] -> w441
          shift-left: "" -> [w444]
          tunnel: [w443] -> w439 mode=indexing
          n246 = Unbundle By Name(w446) -> ("String"=w443:string)
          n247 = Concatenate Strings(w444, w443) -> (w445:string)
        }
        n248 = global write "VAR总磷总氮全局变量.vi" "模块名称"(w441) -> ()
        n249 = property on="单选按钮" class="RadioBtnsControl (严格)"() -> ("Controls[]"=w440:refnum<vi>[])  [unwired: 2 in, 2 out]
        n250 = for {
          tunnel: w440 -> [w454] mode=indexing
          tunnel: w439 -> [w453]
          n251 = property class="Ctl"(reference=w454) -> (reference out=w452:refnum<vi>, "Label.Text"=w448:string)  [unwired: 1 in, 1 out]
          n252 = case shown="\"COD\"" w448 {
            selector: w448 -> [w455 _]
            tunnel: [w455 "CODcr"] -> w447
            frame Default {
            }
            frame "COD" {
            }
          }
          n253 = Search 1D Array(1D array=w453, element=w447) -> (index of element=w451:i32)  [unwired: 1 in]
          n254 = Not Equal?(x=w451, y=-1) -> (x != y?=w449:bool)
          n255 = property class="Ctl"(reference=w452, "Visible"=w449) -> ()  [unwired: 1 in, 2 out]
        }
      }
      frame #1 {
        n256 = Wait (ms)(milliseconds to wait=u32 1000 ("等待时间（毫秒）")) -> ()  [unwired: 1 out]
      }
    }
  }
  n257 = vi-ref "参数设置页.vi"() -> (w16:refnum<vi>)
  n258 = vi-ref "校准设置页.vi"() -> (w12:refnum<vi>)
  n259 = call "时间延迟"("error in (no error)"=w3) -> ("error out"=w25:errorcluster)  [unwired: 10 in]
  n260 = Obtain Notifier(name (unnamed)=w19, notification data type=FALSE) -> (notifier out=w20:refnum<notifier>)  [unwired: 2 in, 2 out]
  n261 = Obtain Queue(name (unnamed)=w19, element data type=cluster{"命令":string, "data":variant} {"命令"="", "data"=variant}) -> (queue out=w22:refnum<queue>)  [unwired: 3 in, 2 out]
  n262 = property class="VI"(reference=w16, error in=w8) -> (reference out=w14:refnum<vi>, "Exec.State"=w15:T13)  [unwired: 1 out]
  n263 = property class="VI"(reference=w12, error in=w7) -> (reference out=w10:refnum<vi>, "Exec.State"=w11:T13)  [unwired: 1 out]
  n264 = while {
    tunnel: w22 -> [w469]
    stop <- FALSE stop-if-true
    n265 = global read "总磷总氮断电保存全局变量.vi" "MB通信方式选择"() -> (w467:enum16{"串口", "TCP"})
    n266 = Get Queue Status(queue=w469) -> (queue out=w468:refnum<queue>, # elements in queue=w464:i32)  [unwired: 2 in, 6 out]
    n267 = global read "VAR总磷总氮全局变量.vi" "MB session in"() -> (w465:refnum<class "MB_Master.lvclass">)
    n268 = global read "VAR总磷总氮全局变量.vi" "升级固件关闭心跳包"() -> (w461:bool)
    n269 = Not(x=w461) -> (.not. x?=w460:bool)
    n270 = case shown="\"串口\", 默认" w467 {
      tunnel: [w472 w473] -> w466
      frame "串口", Default {
        n271 = global read "总磷总氮断电保存全局变量.vi" "VISA Resource"() -> (w472:refnum<visa-resource-name>)
      }
      frame "TCP" {
        n272 = global read "总磷总氮断电保存全局变量.vi" "IP"() -> (w473:string)
      }
    }
    "字符串 2" <- w466
    n273 = property class="MB_Master"(reference=w465) -> ("Properties:Session Valid"=w463:bool)  [unwired: 1 in, 2 out]
    n274 = Equal To 0?(x=w464) -> (x = 0?=w458:bool)
    n275 = Compound Arithmetic op=AND ("复合运算")(w463, w460) -> (w462:bool)
    n276 = global write "VAR总磷总氮全局变量.vi" "心跳包打开状态"(w462) -> ()
    n277 = And(x=w458, y=w462) -> (x .and. y?=w459:bool)
    n278 = case shown="真" w459 {
      tunnel: w468 -> [_ w496]
      frame False {
      }
      frame True {
        n279 = global read "VAR总磷总氮全局变量.vi" "状态告警区"() -> (w489:T6)
        n280 = global read "VAR总磷总氮全局变量.vi" "MB session in"() -> (w483:refnum<class "MB_Master.lvclass">)
        n281 = Unbundle By Name(w489) -> ("系统时间"=w476:timestamp, "工作状态"=w485:u16)
        n282 = property class="MB_Master"(reference=w483) -> ("Properties:Session Valid"=w481:bool)  [unwired: 1 in, 2 out]
        n283 = Get Date/Time In Seconds() -> (seconds since 1Jan1904=w495:timestamp)
        n284 = global read "VAR总磷总氮全局变量.vi" "通讯状态"() -> (w484:bool)
        n285 = case shown="真" w481 {
          tunnel: [_ w498] -> w480
          frame False {
          }
          frame True {
            n286 = global read "VAR总磷总氮全局变量.vi" "MB session in"() -> (w497:refnum<class "MB_Master.lvclass">)
            n287 = call "版本号读取.vi"("MB session in"=w497) -> ("error out"=w498:errorcluster, "固件版本号"=w499:string)  [unwired: 8 in, 1 out]
            "固件版本号" <- w499
            n288 = global write "VAR总磷总氮全局变量.vi" "固件版本号"(w499) -> ()
          }
        }
        n289 = Subtract(x=w495, y=w476) -> (x-y=w494:dbl)
        n290 = Not Equal?(x=w476, y=timestamp(0 s since 1904-01-01)) -> (x != y?=w474:bool)
        n291 = And(x=w481, y=w484) -> (x .and. y?=w482:bool)
        n292 = Absolute Value(x=w494) -> (abs(x)=w493:dbl)
        n293 = Greater Or Equal?(x=w493, y=30.0) -> (x >= y?=w491:bool)
        n294 = global read "VAR总磷总氮全局变量.vi" "通讯状态"() -> (w477:bool)
        n295 = Compound Arithmetic op=AND ("复合运算")(w491, w477, w474) -> (w486:bool)
        n296 = case shown="真" w482 {
          tunnel: [_ w500] -> w479
          tunnel: w480 -> [_ w501]
          frame False {
          }
          frame True {
            n297 = global read "VAR总磷总氮全局变量.vi" "MB session in"() -> (w503:refnum<class "MB_Master.lvclass">)
            n298 = call "序列号读取.vi"("Error in"=w501, "MB session in"=w503) -> ("error out"=w500:errorcluster, "序列号"=w502:string)  [unwired: 7 in, 1 out]
            n299 = global write "VAR总磷总氮全局变量.vi" "序列号"(w502) -> ()
          }
        }
        n300 = Unbundle By Name(w479) -> ("status"=w478:bool)
        n301 = global read "model config var.vi" "启动队列名称"() -> (w487:cluster{"String":string, "Value":u16}[])
        n302 = Not(x=w478) -> ()  [unwired: 1 out]
        n303 = for {
          tunnel: [w521] -> w488 mode=indexing
          tunnel: w487 -> [w522] mode=indexing
          tunnel: w479 -> [_]
          n304 = Unbundle By Name(w522) -> ("Value"=w521:u16)
        }
        n305 = for {
          tunnel: w485 -> [w507]
          shift-right: [w508] -> w490
          shift-left: w496 -> [w510]
          tunnel: w488 -> [w504] mode=indexing
          n306 = Equal?(x=w507, y=T14."空闲") -> (x = y?=w505:bool)
          n307 = Bundle By Name(cluster=cluster{"命令":string, "data":variant} {"命令"="", "data"=variant} ("元素"), "命令"="读状态告警区", "data"=w504) -> (w512:cluster{"命令":string, "data":variant})
          n308 = Enqueue Element(queue=w510, element=w512) -> (queue out=w509:refnum<queue>)  [unwired: 2 in, 2 out]
          n309 = case shown="真" w505 {
            tunnel: w509 -> [w514 w517]
            tunnel: w504 -> [_ w516]
            tunnel: [w514 w515] -> w508
            frame False {
            }
            frame True {
              n310 = Bundle By Name(cluster=cluster{"命令":string, "data":variant} {"命令"="", "data"=variant} ("元素"), "命令"="读测量数据区", "data"=w516) -> (w519:cluster{"命令":string, "data":variant})
              n311 = Enqueue Element(queue=w517, element=w519) -> (queue out=w515:refnum<queue>)  [unwired: 2 in, 2 out]
            }
          }
        }
        n312 = case shown="真" w486 {
          tunnel: w490 -> [_ w524]
          frame False {
          }
          frame True {
            n313 = call "总磷总氮启动命令.vi"("参数"=T15 {"站号"=3, "量程切换"=enum."AUTO", "控制命令"=enum."校时", "模式设置"=enum."待机", "测量间隔"=0}) -> ("启动命令"=w523:cluster{"命令":string, "data":variant})  [unwired: 10 in]
            n314 = Enqueue Element(queue=w524, element=w523) -> ()  [unwired: 2 in, 3 out]
          }
        }
      }
    }
    n315 = Wait (ms)(milliseconds to wait=u32 1000 ("等待时间（毫秒）")) -> ()  [unwired: 1 out]
  }
  n316 = while {
    tunnel: w25 -> [_]
    stop <- FALSE stop-if-true
    n317 = global read "VAR总磷总氮全局变量.vi" "状态告警区"() -> (w557:T6)
    n318 = global read "VAR总磷总氮全局变量.vi" "状态告警区"() -> (w555:T6)
    n319 = global read "VAR总磷总氮全局变量.vi" "状态告警区"() -> (w558:T6)
    n320 = global read "VAR总磷总氮全局变量.vi" "状态告警区"() -> (w559:T6)
    n321 = Unbundle By Name(w557) -> ("flowid"=w528:u16, "工作状态"=w547:u16, "id"=w548:u16)
    n322 = Unbundle By Name(w555) -> ("日志代码"=w554:u16)
    n323 = Unbundle By Name(w558) -> ("日志代码"=w531:u16)
    n324 = Unbundle By Name(w559) -> ("id"=w535:u16, "flowid"=w534:u16, "量程"=w533:u16, "工作状态"=w526:u16, "F0"=→"F0":sgl, "F1"=→"F1":sgl, "F2"=→"F2":sgl, "F3"=→"F3":sgl, "ADC"=→"ADC":sgl, "总磷控温温度1"=→"消解温度":sgl, "营养盐控温温度2"=→"注射器温度":sgl)
    n325 = Not Equal To 0?(x=w547) -> (x != 0?=w545:bool)
    n326 = case shown="0" w547 {
      frame 0 {
        n327 = local write "数组"(string[] [] ("数组")) -> ()
      }
      frame 1, Default {
      }
    }
    n328 = feedback #1(w554) -> (w556:u16)
    n329 = feedback-in #1(w554) -> ()
    n330 = feedback-in #2(w531) -> ()
    n331 = feedback #2(w531) -> (w561:u16)
    n332 = property on="总步数" class="DigNum (严格)"() -> ("Value"=w532:i32)  [unwired: 2 in, 2 out]
    n333 = Subtract(x=w531, y=1) -> (x-y=→"多列列表框":i32)
    n334 = Not Equal?(x=w554, y=w556) -> (x != y?=w553:bool)
    n335 = Not Equal?(x=w531, y=w561) -> (x != y?=w560:bool)
    n336 = Divide(x=w531, y=w532) -> (x/y=w530:dbl)
    n337 = Bundle("id"=w535, "flowid"=w534, "量程"=w533) -> (w536:cluster{"id":u16, "flowid":u16, "量程":u16})  [unwired: 1 in]
    n338 = call <vilib>:"Boolean Crossing PtByPt.vi"("direction"=enum16{"either", "false-true", "true-false"}."false-true", "input"=w545) -> ("crossing"=w549:bool)  [unwired: 1 in]
    n339 = call <vilib>:"Boolean Crossing PtByPt.vi"("direction"=enum16{"either", "false-true", "true-false"}."true-false", "input"=w545) -> ("crossing"=w544:bool)  [unwired: 1 in]
    n340 = case shown="真" w553 {
      frame False {
      }
      frame True {
        n341 = property on="多列列表框" class="MCListbox (严格)"() -> ("ItemNames"=w633:string[][], "Value"=w629:i32)  [unwired: 2 in, 2 out]
        n342 = Index Array(array=w633, index (row)=w629) -> (element=w632:string[])  [unwired: 1 in]
        n343 = Index Array(array=w632) -> (element=w631:string)  [unwired: 1 in]
        n344 = call "过滤筛选流程.vi"("字符串"=w631) -> ("匹配后偏移量"=w630:i32)  [unwired: 10 in]
        n345 = case shown="默认" w630 {
          tunnel: w631 -> [w635 _]
          tunnel: w629 -> [w634 _]
          frame Default {
            n346 = case shown="默认" w635 {
              selector: w635 -> [w641 w648]
              tunnel: [w641 w648] -> w637
              tunnel: [string[] [] ("数组") w643] -> w636
              tunnel: w634 -> [_ w647]
              frame "读数" {
              }
              frame Default {
                n347 = Equal?(x=w647, y=1) -> (x = y?=w645:bool)
                n348 = Select(t=string[] [], s=w645, f="数组") -> (s? t:f=w643:string[])
              }
            }
            n349 = for {
              N: 1 -> [_]
              tunnel: w637 -> [w650]
              shift-right: [w649] -> w638
              shift-left: w636 -> [w651]
              n350 = Search 1D Array(1D array=w651, element=w650) -> (index of element=w654:i32)  [unwired: 1 in]
              n351 = Format Into String(format string="%s" ("格式字符串"), w650) -> (resulting string=w655:string)  [unwired: 2 in, 1 out]
              n352 = Equal?(x=w654, y=-1) -> (x = y?=w652:bool)
              n353 = case shown="真" w652 {
                tunnel: w655 -> [_ w665]
                tunnel: w651 -> [w657 w669]
                tunnel: w650 -> [_ w668]
                tunnel: [w657 w667] -> w649
                frame False {
                }
                frame True {
                  n354 = global read "VAR总磷总氮全局变量.vi" "状态告警区"() -> (w664:T6)
                  n355 = global read "VAR总磷总氮全局变量.vi" "状态告警区"() -> (w679:T6)
                  n356 = global read "VAR总磷总氮全局变量.vi" "状态告警区"() -> (w682:T6)
                  n357 = Insert Into Array(array=w669, new element=w668) -> (w667:string[])  [unwired: 1 in]
                  n358 = Unbundle By Name(w664) -> ("工作状态"=w663:u16, "flowid"=w658:u16)
                  n359 = Unbundle By Name(w679) -> ("F0"=w676:sgl, "F1"=w675:sgl, "F2"=w674:sgl, "F3"=w673:sgl, "id"=w672:u16, "flowid"=w671:u16, "量程"=w670:u16)
                  n360 = Unbundle By Name(w682) -> ("id"=w660:u16)
                  n361 = case shown="2" w663 {
                    selector: w663 -> [w684 _ _ _ _ _ _ _ _ _ _ _]
                    tunnel: [w683 "【水样测试】" ("字符串") w687 "【零点核查】" ("字符串") "【跨度核查】" ("字符串") "【空白测试】" ("字符串") "【平行样测试】" ("字符串") "【加标回收】" ("字符串") "【空白校准】" ("字符串") "【标样校准】" ("字符串") "【单步调试】" ("字符串") w698] -> w661
                    tunnel: w658 -> [_ _ w686 _ _ _ _ _ _ _ _ _]
                    frame 0, Default {
                      n362 = Number To Decimal String(number=w684) -> (decimal integer string=w683:string)  [unwired: 1 in]
                    }
                    frame 1 {
                    }
                    frame 2 {
                      n363 = case shown="5" w686 {
                        tunnel: ["【标样核查】" ("字符串") "【快捷测试】" ("字符串")] -> w687
                        frame Default {
                        }
                        frame 5 {
                        }
                      }
                    }
                    frame 3 {
                    }
                    frame 4 {
                    }
                    frame 5 {
                    }
                    frame 6 {
                    }
                    frame 7 {
                    }
                    frame 8 {
                    }
                    frame 9 {
                    }
                    frame 254 {
                    }
                    frame 255 {
                      n364 = local read "简易步骤名称"() -> (w700:string)
                      n365 = Format Into String(format string="(%s)" ("格式字符串"), initial string="【简易流程】" ("工作状态"), w700) -> (resulting string=w698:string)  [unwired: 1 in, 1 out]
                    }
                  }
                  n366 = call "id参数转换.vi"("id"=w660) -> ("table输出"=w659:string)  [unwired: 9 in, 1 out]
                  n367 = Format Into String(format string="F0=%#f,F1=%#f,F2=%#f,F3=%#f,Flow=%d-%-d-%-d" ("格式字符串"), w676, w675, w674, w673, w672, w671, w670) -> (resulting string=w677:string)  [unwired: 2 in, 1 out]
                  n368 = Concatenate Strings(w661, w665) -> (w662:string)
                  n369 = Get Date/Time In Seconds() -> (seconds since 1Jan1904=w680:timestamp)
                  n370 = Bundle By Name(cluster=T16 {"时间标识"=timestamp(0 s since 1904-01-01), "设备"="", "日志信息"="", "流程参数"=""} ("data in"), "时间标识"=w680, "设备"=w659, "日志信息"=w662, "流程参数"=w677) -> (w681:T16)
                  n371 = call "总磷总氮操作日志.vi"("data in"=w681) -> ()  [unwired: 10 in, 1 out]
                }
              }
            }
            n372 = local write "数组"(w638) -> ()
          }
          frame -1 {
          }
        }
      }
    }
    n373 = case shown="真" w560 {
      tunnel: w531 -> [_ w735]
      frame False {
      }
      frame True {
        n374 = Subtract(x=w735, y=1) -> (x-y=w733:i32)
        n375 = Subtract(x=w733, y=5) -> (x-y=w737:i32)
        n376 = Greater Or Equal To 0?(x=w737) -> (x >= 0?=w736:bool)
        n377 = property on="多列列表框" class="MCListbox (严格)"() -> (error out=w741:errorcluster, "TopLeft"=w742:T17)  [unwired: 2 in, 1 out]
        n378 = Select(t=w737, s=w736, f=0) -> (s? t:f=w738:i32)
        n379 = Bundle By Name(cluster=w742, "Row"=w738) -> (w743:T17)
        n380 = property on="多列列表框" class="MCListbox (严格)"(error in=w741, "TopLeft"=w743) -> ()  [unwired: 1 in, 2 out]
      }
    }
    n381 = while {
      tunnel: w536 -> [w717]
      shift-right: [w713] -> _
      shift-left: _ -> [w714]
      shift-right: [w706] -> _
      shift-left: _ -> [w715]
      shift-right: [w707] -> _
      shift-left: _ -> [w712]
      shift-right: [w703] -> _
      shift-left: _ -> [w710]
      tunnel: w526 -> [w703]
      stop <- TRUE stop-if-true
      n382 = Not Equal?(x=w710, y=w703) -> (x != y?=w709:bool)
      n383 = case shown="255" w703 {
        tunnel: [w718 w719] -> w707
        frame 0, Default {
          n384 = global read "总磷总氮断电保存全局变量.vi" "流程路径"() -> (w718:path)
        }
        frame 255 {
          n385 = global read "总磷总氮断电保存全局变量.vi" "简易流程路径"() -> (w719:path)
        }
      }
      n386 = Not Equal To 0?(x=w703) -> (x != 0?=w702:bool)
      n387 = Not Equal?(x=w712, y=w707) -> (x != y?=w708:bool)
      n388 = Compound Arithmetic op=OR ("复合运算")(w708, w709) -> (w711:bool)
      n389 = And(x=w702, y=w711) -> (x .and. y?=w704:bool)
      n390 = case shown="真" w704 {
        tunnel: [w721 w731] -> w706
        tunnel: [w720 w730] -> w713
        tunnel: w717 -> [_ w725]
        tunnel: w715 -> [w721 _]
        tunnel: w714 -> [w720 _]
        tunnel: w707 -> [_ w724]
        tunnel: w703 -> [_ w723]
        frame False {
        }
        frame True {
          n391 = call "斯坦道XML解析.vi"("工作状态"=w723, "添加的路径"=w724, "参数簇"=w725) -> ("简易步骤名称"=→"简易步骤名称":string, "步骤时间"=w726:string[], "步骤名"=w728:string[])  [unwired: 6 in]
          n392 = for {
            tunnel: w728 -> [_] mode=indexing
            tunnel: [w732] -> w729 mode=indexing
            i -> [w732]
          }
          n393 = Build Array(w728, w726) -> (w727:string[][])
          n394 = Transpose 2D Array(2D array=w727) -> (transposed array=w730:string[][])
          n395 = Number To Decimal String(number=w729) -> (decimal integer string=w731:string[])  [unwired: 1 in]
        }
      }
      n396 = property on="多列列表框" class="MCListbox (严格)"("ItemNames"=w713, "RowHdrs[]"=w706) -> ()  [unwired: 2 in, 2 out]
      n397 = Array Size(array=w706) -> (size(s)=→"总步数":i32)
    }
    n398 = Multiply(x=w530, y=100.0) -> (x*y=w527:dbl)
    "滑动杆" <- w527
    n399 = case shown="真" w549 {
      tunnel: w547 -> [_ w606]
      tunnel: w548 -> [_ w603]
      tunnel: w528 -> [_ w601]
      frame False {
      }
      frame True {
        n400 = case shown="8" w606 {
          selector: w606 -> [w613 _ _ _ _ _ _ _ _ _ _ _]
          tunnel: [w612 "【水样测试】" ("字符串") w616 "【零点核查】" ("字符串") "【跨度核查】" ("字符串") "【空白测试】" ("字符串") "【平行样测试】" ("字符串") "【加标回收】" ("字符串") "【空白校准】" ("字符串") "【标样校准】" ("字符串") "【单步调试】" ("字符串") "【简易流程】" ("字符串")] -> w611
          tunnel: w601 -> [_ _ w615 _ _ _ _ _ _ _ _ _]
          frame 0, Default {
            n401 = Number To Decimal String(number=w613) -> (decimal integer string=w612:string)  [unwired: 1 in]
          }
          frame 1 {
          }
          frame 2 {
            n402 = case shown="5" w615 {
              tunnel: ["【标样核查】" ("字符串") "【快捷测试】" ("字符串")] -> w616
              frame 0, Default {
              }
              frame 5 {
              }
            }
          }
          frame 3 {
          }
          frame 4 {
          }
          frame 5 {
          }
          frame 6 {
          }
          frame 7 {
          }
          frame 8 {
          }
          frame 9 {
          }
          frame 254 {
          }
          frame 255 {
          }
        }
        n403 = call "id参数转换.vi"("id"=w603) -> ("table输出"=w602:string)  [unwired: 9 in, 1 out]
        n404 = Concatenate Strings("<<" ("字符串"), w611, "启动" ("字符串")) -> (w610:string)
        n405 = Get Date/Time In Seconds() -> (seconds since 1Jan1904=w608:timestamp)
        n406 = Bundle By Name(cluster=T16 {"时间标识"=timestamp(0 s since 1904-01-01), "设备"="", "日志信息"="", "流程参数"=""} ("data in"), "时间标识"=w608, "设备"=w602, "日志信息"=w610) -> (w607:T16)
        n407 = call "总磷总氮操作日志.vi"("data in"=w607) -> ()  [unwired: 10 in, 1 out]
      }
    }
    n408 = case shown="真" w544 {
      tunnel: w548 -> [_ w579]
      tunnel: w528 -> [_ w565]
      frame False {
      }
      frame True {
        n409 = global read "VAR总磷总氮全局变量.vi" "最近一次工作状态"() -> (w564:u16)
        n410 = global read "VAR总磷总氮全局变量.vi" "状态告警区"() -> (w577:T6)
        n411 = call "id参数转换.vi"("id"=w579) -> ("table输出"=w578:string)  [unwired: 9 in, 1 out]
        n412 = case shown="2" w564 {
          selector: w564 -> [w586 _ _ _ _ _ _ _ _ _ _ _]
          tunnel: [w585 "【水样测试】" ("字符串") w589 "【零点核查】" ("字符串") "【跨度核查】" ("字符串") "【空白测试】" ("字符串") "【平行样测试】" ("字符串") "【加标回收】" ("字符串") "【空白校准】" ("字符串") "【标样校准】" ("字符串") "【单步调试】" ("字符串") "【简易流程】" ("字符串")] -> w567
          tunnel: w565 -> [_ _ w588 _ _ _ _ _ _ _ _ _]
          frame 0, Default {
            n413 = Number To Decimal String(number=w586) -> (decimal integer string=w585:string)  [unwired: 1 in]
          }
          frame 1 {
          }
          frame 2 {
            n414 = case shown="0, 默认" w588 {
              tunnel: ["【标样核查】" ("字符串") "【快捷测试】" ("字符串")] -> w589
              frame 0, Default {
              }
              frame 5 {
              }
            }
          }
          frame 3 {
          }
          frame 4 {
          }
          frame 5 {
          }
          frame 6 {
          }
          frame 7 {
          }
          frame 8 {
          }
          frame 9 {
          }
          frame 254 {
          }
          frame 255 {
          }
        }
        n415 = Unbundle By Name(w577) -> ("F0"=w576:sgl, "F1"=w575:sgl, "F2"=w574:sgl, "F3"=w573:sgl, "id"=w572:u16, "flowid"=w571:u16, "量程"=w570:u16)
        n416 = Format Into String(format string="F0=%#f,F1=%#f,F2=%#f,F3=%#f,Flow=%d-%-d-%-d" ("格式字符串"), w576, w575, w574, w573, w572, w571, w570) -> (resulting string=w568:string)  [unwired: 2 in, 1 out]
        n417 = Concatenate Strings(w567, "停止" ("字符串"), ">>" ("字符串")) -> (w584:string)
        n418 = Get Date/Time In Seconds() -> (seconds since 1Jan1904=w582:timestamp)
        n419 = Bundle By Name(cluster=T16 {"时间标识"=timestamp(0 s since 1904-01-01), "设备"="", "日志信息"="", "流程参数"=""} ("data in"), "时间标识"=w582, "设备"=w578, "日志信息"=w584, "流程参数"=w568) -> (w581:T16)
        n420 = call "总磷总氮操作日志.vi"("data in"=w581) -> ()  [unwired: 10 in, 1 out]
      }
    }
    n421 = global write "VAR总磷总氮全局变量.vi" "测试进度"(w527) -> ()
    n422 = Wait (ms)(milliseconds to wait=u32 1000 ("等待时间（毫秒）")) -> ()  [unwired: 1 out]
  }
  n423 = case shown="\"Bad\", 默认" w15 {
    tunnel: w14 -> [w744 w748]
    tunnel: [w744 w745] -> w13
    frame "Bad", Default {
    }
    frame "Idle" {
      n424 = invoke class="VI" method="Run VI"(reference=w748, "Wait until done"=FALSE ("结束前等待"), "Auto Dispose Ref"=TRUE ("自动销毁引用")) -> (reference out=w745:refnum<vi>)  [unwired: 2 in, 4 out]
    }
  }
  n425 = case shown="\"Bad\", 默认" w11 {
    tunnel: w10 -> [w749 w753]
    tunnel: [w749 w750] -> w9
    frame "Bad", Default {
    }
    frame "Idle" {
      n426 = invoke class="VI" method="Run VI"(reference=w753, "Wait until done"=FALSE ("结束前等待"), "Auto Dispose Ref"=TRUE ("自动销毁引用")) -> (reference out=w750:refnum<vi>)  [unwired: 2 in, 4 out]
    }
  }
  n427 = while {
    tunnel: w22 -> [w757]
    tunnel: w20 -> [w756]
    tunnel: w13 -> [w755]
    tunnel: w9 -> [w754]
    stop <- FALSE stop-if-true
    n428 = event shown="[10] \"停止\": 值改变" {
      selector: _ -> [_ _ _ _ _ _ _ _ _ _ _ _ _ _]
      dyn-events: _ -> [_ _ _ _ _ _ _ _ _ _ _ _ _ _]
      timeout: _ -> [_ _ _ _ _ _ _ _ _ _ _ _ _ _]
      tunnel: w757 -> [_ _ _ _ _ _ _ _ w771 _ w778 _ _ _]
      tunnel: w756 -> [_ _ _ _ _ _ _ _ _ _ w777 _ _ _]
      tunnel: w755 -> [_ _ _ _ _ _ _ _ _ _ _ w798 _ _]
      tunnel: w754 -> [_ _ _ _ _ _ _ _ _ _ _ _ w804 _]
      event Timeout {
        n429 = event-data() -> ()  [unwired: 1 in, 3 out]
      }
      event "流程操作": Value Change {
        n430 = event-data() -> ()  [unwired: 1 in, 6 out]
        n431 = global read "总磷总氮断电保存全局变量.vi" "流程路径"() -> (w760:path)
        n432 = global read "总磷总氮断电保存全局变量.vi" "简易流程路径"() -> (w759:path)
        n433 = call "流程批量写入.vi"("简易流程路径"=w759, "添加的路径"=w760) -> ()  [unwired: 10 in]
      }
      event "温度曲线": Value Change {
        n434 = event-data() -> ()  [unwired: 1 in, 6 out]
        n435 = call "温度曲线显示.vi"() -> ()  [unwired: 12 in]
      }
      event "试剂余量": Value Change {
        n436 = event-data() -> ()  [unwired: 1 in, 6 out]
        n437 = call "试剂余量显示UI.vi"() -> ()  [unwired: 12 in]
      }
      event "灯值调整": Value Change {
        n438 = event-data() -> ()  [unwired: 1 in, 6 out]
        n439 = call "灯值调整对话框.vi"() -> ()  [unwired: 12 in]
      }
      event "布尔": Value Change {
        n440 = event-data() -> ("NewVal"=w761:bool)  [unwired: 1 in, 5 out]
        n441 = case shown="假" w761 {
          frame False {
            n442 = global write "VAR总磷总氮全局变量.vi" "权限等级"(enum16{"一级权限", "二级权限", "三级权限", "超级权限"}."一级权限" ("权限等级")) -> ()
          }
          frame True {
            n443 = global read "VAR总磷总氮全局变量.vi" "权限密码"() -> (w765:u32[])
            n444 = global read "VAR总磷总氮全局变量.vi" "权限等级"() -> (w763:enum16{"一级权限", "二级权限", "三级权限", "超级权限"})
            n445 = call "密码权限设置.vi"("权限输入"=w763, "权限密码"=w765) -> ("权限输出"=w764:enum16{"一级权限", "二级权限", "三级权限", "超级权限"})  [unwired: 9 in]
            n446 = global write "VAR总磷总氮全局变量.vi" "权限等级"(w764) -> ()
          }
        }
      }
      event "权限等级": Mouse Down {
        n447 = event-data() -> ()  [unwired: 1 in, 8 out]
        n448 = global read "VAR总磷总氮全局变量.vi" "权限密码"() -> (w768:u32[])
        n449 = global read "VAR总磷总氮全局变量.vi" "权限等级"() -> (w766:enum16{"一级权限", "二级权限", "三级权限", "超级权限"})
        n450 = call "密码权限设置.vi"("权限输入"=w766, "权限密码"=w768) -> ("权限输出"=w767:enum16{"一级权限", "二级权限", "三级权限", "超级权限"})  [unwired: 9 in]
        n451 = global write "VAR总磷总氮全局变量.vi" "权限等级"(w767) -> ()
      }
      event "外设固件": Value Change {
        n452 = event-data() -> ()  [unwired: 1 in, 6 out]
        n453 = call "流程固件设置对话框.vi"() -> ()  [unwired: 12 in]
      }
      event "手动启动": Value Change {
        n454 = event-data() -> ()  [unwired: 1 in, 6 out]
        n455 = call "总磷总氮启动参数对话框.vi"() -> ("确认"=w769:bool, "元素"=w770:cluster{"命令":string, "data":variant})  [unwired: 10 in]
        n456 = case shown="真" w769 {
          tunnel: w771 -> [_ w774]
          tunnel: w770 -> [_ w773]
          frame False {
          }
          frame True {
            n457 = Flush Queue(queue=w774) -> (queue out=w772:refnum<queue>)  [unwired: 1 in, 2 out]
            n458 = Enqueue Element(queue=w772, element=w773) -> ()  [unwired: 2 in, 3 out]
          }
        }
      }
      event "调试": Value Change {
        n459 = event-data() -> ()  [unwired: 1 in, 6 out]
        n460 = call "简易流程调试界面.vi"() -> ()  [unwired: 12 in]
      }
      event "停止": Value Change {
        n461 = event-data() -> ()  [unwired: 1 in, 6 out]
        n462 = Two Button Dialog(message="确认停止？" ("消息")) -> (T button?=w775:bool)  [unwired: 2 in]
        n463 = case shown="真" w775 {
          tunnel: w778 -> [_ w794]
          tunnel: w777 -> [_ w793]
          frame False {
          }
          frame True {
            n464 = global read "VAR总磷总氮全局变量.vi" "状态告警区"() -> (w780:T6)
            n465 = global read "VAR总磷总氮全局变量.vi" "状态告警区"() -> (w788:T6)
            n466 = Send Notification(notification=TRUE ("通知"), notifier=w793) -> ()  [unwired: 1 in, 2 out]
            n467 = Unbundle By Name(w780) -> ("id"=w779:u16)
            n468 = Unbundle By Name(w788) -> ("id"=w787:u16)
            n469 = call "id参数转换.vi"("id"=w779) -> ("table输出"=w781:string)  [unwired: 9 in, 1 out]
            n470 = Bundle By Name(cluster=T15 {"站号"=1, "量程切换"=enum."AUTO", "控制命令"=enum."停止测试", "模式设置"=enum."待机", "测量间隔"=0} ("参数"), "站号"=w787) -> (w789:T15)
            n471 = Get Date/Time In Seconds() -> (seconds since 1Jan1904=w784:timestamp)
            n472 = call "总磷总氮启动命令.vi"("参数"=w789) -> ("启动命令"=w790:cluster{"命令":string, "data":variant})  [unwired: 10 in]
            n473 = Bundle By Name(cluster=T18 {"时间"=timestamp(0 s since 1904-01-01), "参数"="", "日志信息"="", "流程参数"=""} ("data in"), "时间"=w784, "参数"=w781, "日志信息"="手动停止") -> (w785:T18)
            n474 = Enqueue Element(queue=w794, element=w790) -> (error out=w782:errorcluster)  [unwired: 2 in, 2 out]
            n475 = call "总磷总氮操作日志.vi"("错误输入（无错误）"=w782, "data in"=w785) -> ()  [unwired: 9 in, 1 out]
          }
        }
      }
      event "参数设置", "参数查询": Value Change {
        n476 = event-data() -> ()  [unwired: 1 in, 6 out]
        n477 = invoke on="子面板" class="SubPnl" method="Remove VI"() -> (error out=w799:errorcluster)  [unwired: 3 in, 2 out]
        n478 = global write "VAR总磷总氮全局变量.vi" "页面"(enum16{"主页", "参数页", "校准页"}."参数页" ("页面")) -> ()
        n479 = property on="仪器校准" class="Bool"("Visible"=TRUE ("可见")) -> ()  [unwired: 2 in, 2 out]
        n480 = property on="参数查询" class="Bool"("Visible"=FALSE ("可见")) -> ()  [unwired: 2 in, 2 out]
        n481 = invoke on="子面板" class="SubPnl" method="Insert VI"(error in=w799, "VI Ref"=w798) -> ()  [unwired: 2 in, 4 out]
        n482 = property on="窗格" class="Pane"("Origin"=T5 {"Horizontal"=0, "Vertical"=640} ("原点")) -> ()  [unwired: 2 in, 2 out]
      }
      event "仪器校准": Value Change {
        n483 = event-data() -> ()  [unwired: 1 in, 6 out]
        n484 = invoke on="子面板" class="SubPnl" method="Remove VI"() -> (error out=w805:errorcluster)  [unwired: 3 in, 2 out]
        n485 = global write "VAR总磷总氮全局变量.vi" "页面"(enum16{"主页", "参数页", "校准页"}."校准页" ("页面")) -> ()
        n486 = property on="仪器校准" class="Bool"("Visible"=FALSE ("可见")) -> ()  [unwired: 2 in, 2 out]
        n487 = invoke on="子面板" class="SubPnl" method="Insert VI"(error in=w805, "VI Ref"=w804) -> ()  [unwired: 2 in, 4 out]
        n488 = property on="参数查询" class="Bool"("Visible"=TRUE ("可见")) -> ()  [unwired: 2 in, 2 out]
      }
      event "返回": Value Change {
        n489 = event-data() -> ()  [unwired: 1 in, 6 out]
        n490 = global write "VAR总磷总氮全局变量.vi" "页面"(enum16{"主页", "参数页", "校准页"}."主页" ("页面")) -> ()
        n491 = property on="窗格" class="Pane"("Origin"=T5 {"Horizontal"=0, "Vertical"=0} ("原点")) -> ()  [unwired: 2 in, 2 out]
      }
    }
  }
